vi "PwF_ToF_FlashLED.vi"(0 "HW Serial Number":u32=255, 11 "error in (no error)":errorcluster) -> (15 "error out":errorcluster)   [LabVIEW 2018]
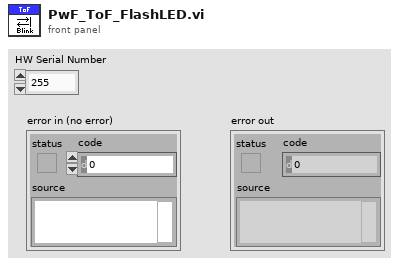
[diagram p1: front panel]
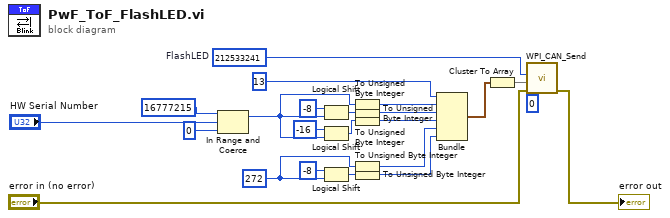
[diagram p0: block diagram]
diagram:
  w5 = u16 272 ("y")
  w16 = u32 212533241  # FlashLED
  n1 = In Range and Coerce(upper limit=u32 16777215, x="HW Serial Number", lower limit=u32 0) -> (coerced(x)=w10:u32)  [unwired: 1 out]
  n2 = Logical Shift(y=i16 -8, x=w10) -> (x << y=w22:u32)
  n3 = Logical Shift(y=i16 -16, x=w10) -> (x << y=w9:u32)
  n4 = Logical Shift(y=i16 -8, x=w5) -> (x << y=w6:u16)
  n5 = To Unsigned Byte Integer(number=w10) -> (unsigned 8bit integer=w21:u8)
  n6 = To Unsigned Byte Integer(number=w22) -> (unsigned 8bit integer=w20:u8)
  n7 = To Unsigned Byte Integer(number=w9) -> (unsigned 8bit integer=w8:u8)
  n8 = To Unsigned Byte Integer(number=w5) -> (unsigned 8bit integer=w4:u8)
  n9 = To Unsigned Byte Integer(number=w6) -> (unsigned 8bit integer=w3:u8)
  n10 = Bundle("y"=u8 13, w21, w20, w8, w4, w3) -> (w2:cluster{"y":u8, u8, u8, u8, u8, u8})  [unwired: 1 in]
  n11 = Cluster To Array(cluster=w2) -> (array=w1:u8[])
  n12 = call <vilib>:"WPI_CAN_Send.vi"("Period (ms)"=0, "error in (no error)"="error in (no error)", "Data"=w1, "Message ID"=w16) -> ("error out"=→"error out":errorcluster)  [unwired: 7 in]
